vi "PI Controller.vi"(1 "Sampling time":dbl, 2 "PI Parameter":T1, 3 "Reference Value [Celsius]":dbl, 4 "Process Value [Celsius]":dbl) -> (0 "Control Value (u)":dbl)   [LabVIEW 2023]
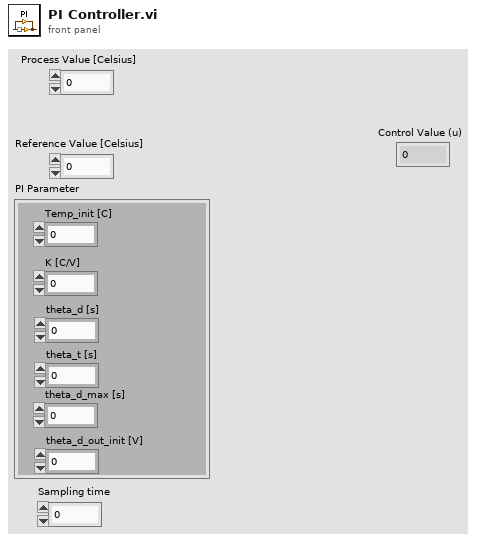
[diagram p1: front panel]
types:
  T1 = cluster{"theta_d_max [s]":dbl, "theta_d_out_init [V]":dbl, "theta_t [s]":dbl, "theta_d [s]":dbl, "K [C/V]":dbl, "Temp_init [C]":dbl}
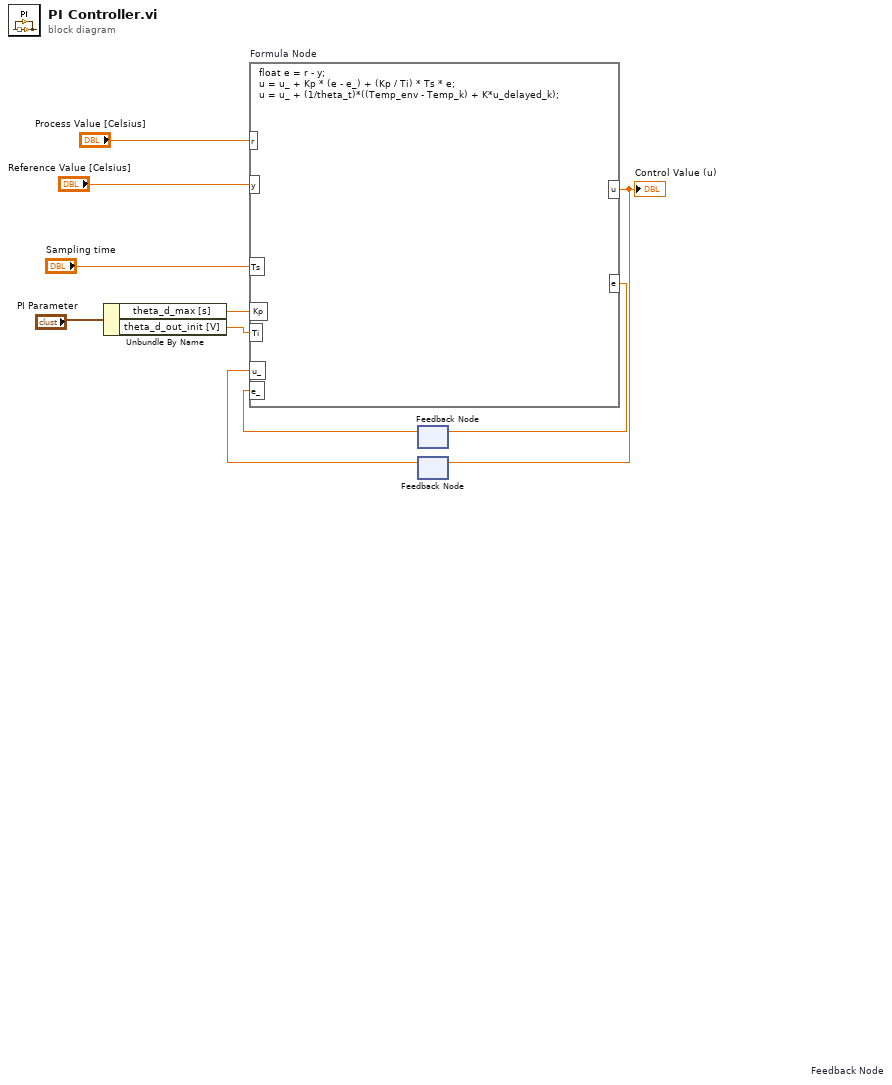
[diagram p0: block diagram]
diagram:
  n1 = Unbundle By Name("PI Parameter") -> ("theta_d_max [s]"=w7:dbl, "theta_d_out_init [V]"=w8:dbl)
  n2 = feedback #1() -> (w2:dbl)  [unwired: 1 in]
  n3 = feedback #2 "Feedback Node"() -> (w4:dbl)  [unwired: 1 in]
  n4 = formula code="float e = r - y;\nu = u_ + Kp * (e - e_) + (Kp / Ti) * Ts * e;\nu = u_ + (1/theta_t)*((Temp_env - Temp_k) + K*u_delayed_k);"("r"="Process Value [Celsius]", "y"="Reference Value [Celsius]", "Kp"=w7, "Ti"=w8, "Ts"="Sampling time", "u_"=w4, "e_"=w2) -> ("u"=w5:dbl, "e"=w3:dbl)
  "Control Value (u)" <- w5
  n5 = feedback-in #1(w3) -> ()
  n6 = feedback-in #2(w5) -> ()
